vi "Unpack Zip.vi"(8 "error in (no error)":errorcluster, 11 "Zip":path) -> (0 "error out":errorcluster, 2 "Solver VI":path, 3 "Folder":path)   [LabVIEW 2024, in "Word Search Scorer.lvlib"]
uses:
  Word Search Scorer.lvlib
  <vilib>/zip/NI_Unzip.lvlib
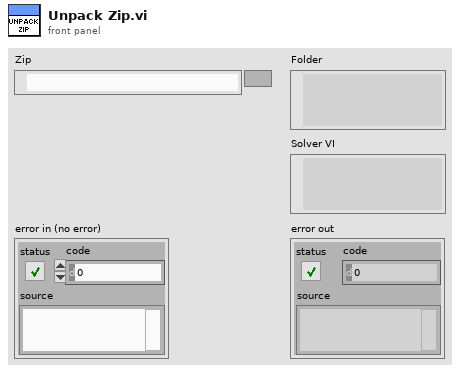
[diagram p1: front panel]
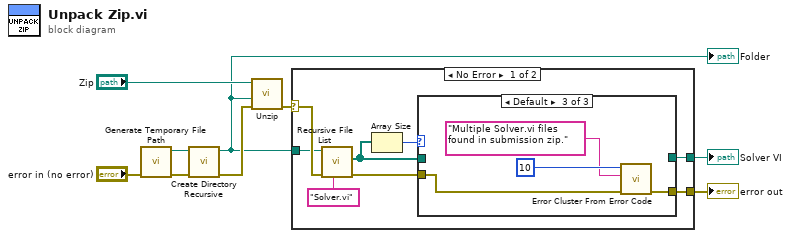
[diagram p0: block diagram]
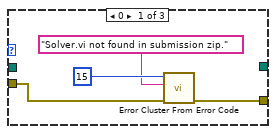
[diagram p2: hidden frame]
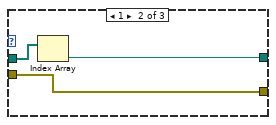
[diagram p3: hidden frame]
diagram:
  n1 = call <vilib>:"Generate Temporary File Path.vi"("error in (no error)"="error in (no error)") -> ("error out"=w6:errorcluster, "Unique Temporary File Path"=w7:path)  [unwired: 9 in]
  n2 = call <vilib>:"Create Directory Recursive.vi"("error in (no error)"=w6, "directory"=w7) -> ("error out"=w5:errorcluster, "directory copy"=w3:path)  [unwired: 3 in, 1 out]
  "Folder" <- w3
  n3 = call <vilib>:"Unzip.vi"("error in (no error)"=w5, "Target directory (same as Zip file if empty)"=w3, "Zip file"="Zip") -> ("error out"=w1:errorcluster)  [unwired: 6 in, 2 out]
  n4 = case shown="No Error" w1 {
    selector: w1 -> [w17 _]
    tunnel: w3 -> [w16 _]
    tunnel: [w11 _] -> w2
    tunnel: [w10 _] -> w9
    frame No Error {
      n5 = call <vilib>:"Recursive File List.vi"("pattern"="Solver.vi", "error in (no error)"=w17, "Folder Path"=w16) -> ("error out"=w12:errorcluster, "All Files in Dir"=w13:path[])  [unwired: 4 in, 3 out]
      n6 = Array Size(array=w13) -> (size(s)=w14:i32)
      n7 = case shown="Default" w14 {
        tunnel: w13 -> [_ w24 _]
        tunnel: w12 -> [w21 w22 w27]
        tunnel: [_ w23 _] -> w11
        tunnel: [w18 w22 w28] -> w10
        frame 0 {
          n8 = call <vilib>:"Error Cluster From Error Code.vi"("error in (no error)"=w21, "error message (\"\")"="Solver.vi not found in submission zip.", "error code (0)"=15) -> ("error out"=w18:errorcluster)  [unwired: 6 in]
        }
        frame 1 {
          n9 = Index Array(array=w24) -> (element=w23:path)  [unwired: 1 in]
        }
        frame Default {
          n10 = call <vilib>:"Error Cluster From Error Code.vi"("error in (no error)"=w27, "error message (\"\")"="Multiple Solver.vi files found in submission zip.", "error code (0)"=10) -> ("error out"=w28:errorcluster)  [unwired: 6 in]
        }
      }
    }
    frame Error {
    }
  }
  "error out" <- w9
  "Solver VI" <- w2
